vi "WebView2 Demo Browser.vi"() -> ()   [LabVIEW 2020]
uses:
  Webview2 Control/WebView2 Control.xctl
  Webview2 Control/Paths.ctl
panel:
  out "Paths":T1
  in  "stop":bool
  in  "FWD":bool
  in  "Back":bool
  out "Status":string
  out "navigation complete":bool
  in  "Reload":bool
  in  "Go":bool
  in  "URL":string="http://ni.com"
  out "WebView2 Browser Control":string(xcontrol)
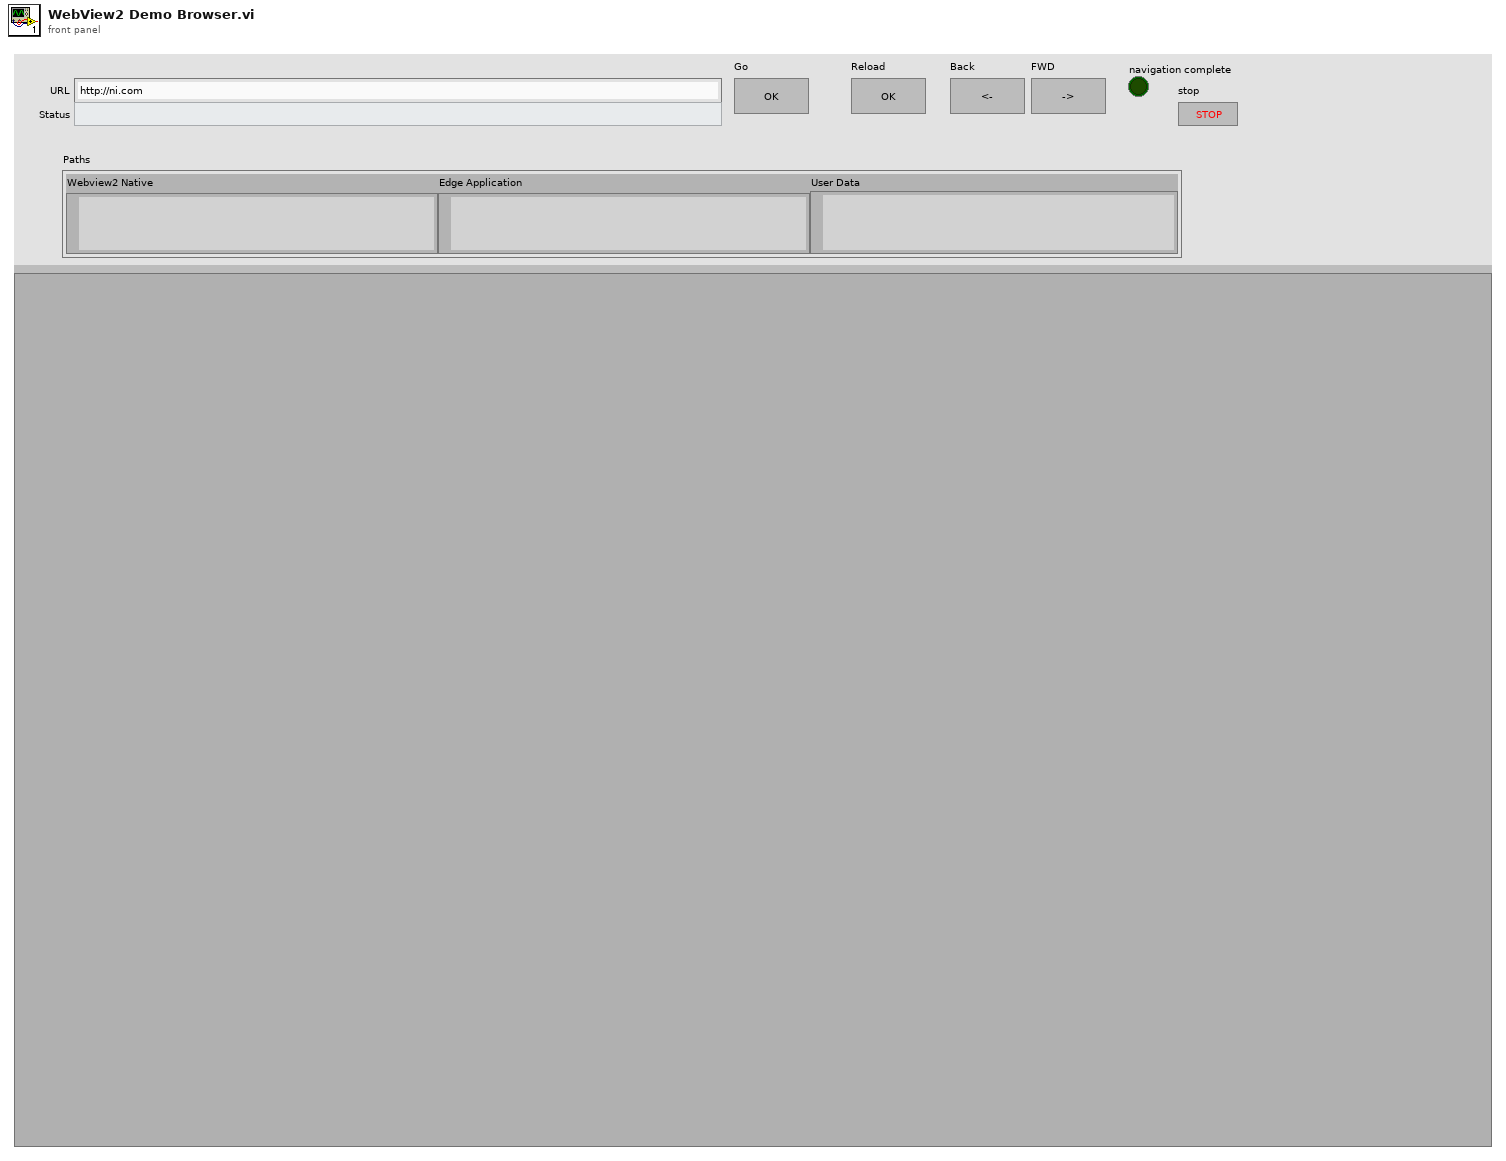
[diagram p1: front panel]
types:
  T1 = typedef "WebView2 Control.xctl/Paths.ctl" = cluster{"Webview2 Native":path, "Edge Application":path, "User Data":path}
  T2 = cluster{"Navigation Complete Event":refnum<user-event>, "Source Changed Event":refnum<user-event>, "Document Title Changed Event":refnum<user-event>, "Status Bar Text Changed":refnum<user-event>, "Web Message Received":refnum<user-event>, "Window Close Requested":refnum<user-event>}
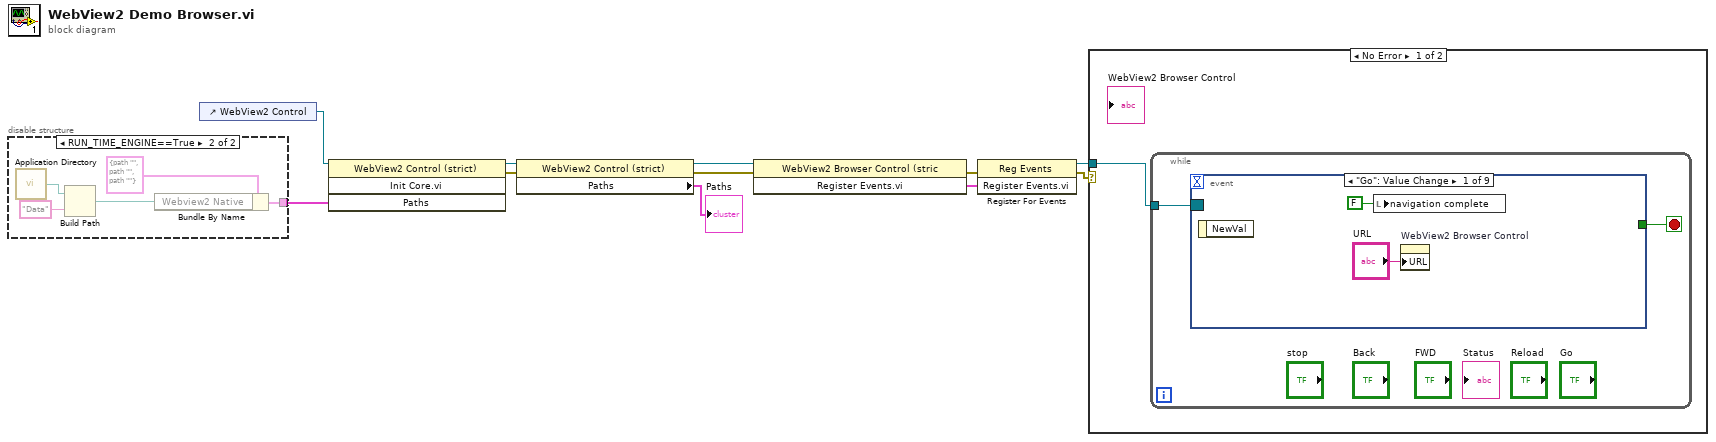
[diagram p0: block diagram]
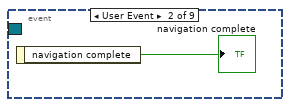
[diagram p3: hidden frame]
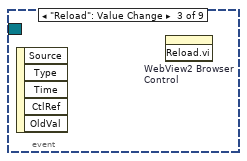
[diagram p4: hidden frame]
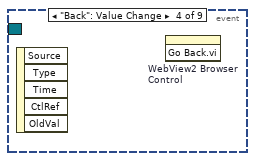
[diagram p5: hidden frame]
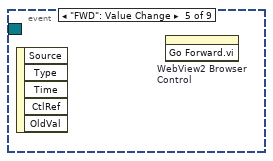
[diagram p6: hidden frame]
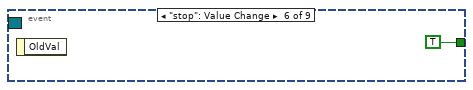
[diagram p7: hidden frame]
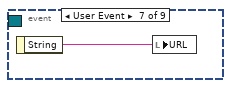
[diagram p8: hidden frame]
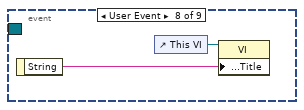
[diagram p9: hidden frame]
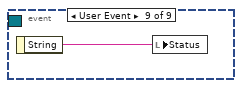
[diagram p10: hidden frame]
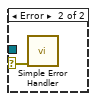
[diagram p11: hidden frame]
diagram:
  n1 = disable-structure shown="RUN_TIME_ENGINE==True" {
    disable-tunnel: [_ w15] -> w1
    frame condition #0 (active) {
    }
    frame condition #1 {
      n2 = call <vilib>:"Application Directory.vi"() -> ("Application Directory"=w13:path)
      n3 = Build Path(base path=w13, name or relative path="Data") -> (appended path=w14:path)
      n4 = Bundle By Name(cluster=T1 {"Webview2 Native"=path "", "Edge Application"=path "", "User Data"=path ""} ("Path Overrides"), "Webview2 Native"=w14) -> (w15:T1)
    }
  }
  n5 = control-ref of="WebView2 Control"() -> (w4:refnum<vi>)
  n6 = invoke class="WebView2 Control (strict)" method="Init Core.vi"(reference=w4, "Paths"=w1) -> (reference out=w3:refnum<vi>, error out=w2:errorcluster)  [unwired: 2 in, 2 out]
  n7 = property class="WebView2 Control (strict)"(reference=w3, error in=w2) -> (reference out=w9:refnum<vi>, error out=w8:errorcluster, "Paths"=→"Paths":T1)
  n8 = invoke class="WebView2 Browser Control (stric" method="Register Events.vi"(reference=w9, error in=w8) -> (error out=w6:errorcluster, "Register Events.vi"=w5:T2)  [unwired: 1 in, 1 out]
  n9 = register-events(error in=w6, w5) -> (reference out=w11:refnum<event-registration>, error out=w10:errorcluster)  [unwired: 1 in]
  n10 = case shown="No Error" w10 {
    selector: w10 -> [_ w28]
    tunnel: w11 -> [w17 _]
    frame No Error {
      n11 = while {
        tunnel: w17 -> [w19]
        stop <- w18 stop-if-true
        n12 = event shown="[0] \"Go\": Value Change" {
          selector: w19 -> [_ _ _ _ _ _ _ _ _]
          dyn-events: _ -> [_ _ _ _ _ _ _ _ _]
          timeout: _ -> [_ _ _ _ _ _ _ _ _]
          tunnel: [_ _ _ _ _ TRUE _ _ _] -> w18
          event "Go": Value Change {
            n13 = event-data() -> ()  [unwired: 1 in, 1 out]
            n14 = local write "navigation complete"(FALSE ("navigation complete")) -> ()
            n15 = property on="WebView2 Browser Control" class="WebView2 Control (strict)"("URL"="URL") -> ()  [unwired: 2 in, 2 out]
          }
          event User Event {
            n16 = event-data() -> ("navigation complete"=→"navigation complete":bool)  [unwired: 1 in]
          }
          event "Reload": Value Change {
            n17 = event-data() -> ()  [unwired: 1 in, 5 out]
            n18 = invoke on="WebView2 Browser Control" class="WebView2 Browser Control (stric" method="Reload.vi"() -> ()  [unwired: 3 in, 3 out]
          }
          event "Back": Value Change {
            n19 = event-data() -> ()  [unwired: 1 in, 5 out]
            n20 = invoke on="WebView2 Browser Control" class="WebView2 Browser Control (stric" method="Go Back.vi"() -> ()  [unwired: 3 in, 3 out]
          }
          event "FWD": Value Change {
            n21 = event-data() -> ()  [unwired: 1 in, 5 out]
            n22 = invoke on="WebView2 Browser Control" class="WebView2 Browser Control (stric" method="Go Forward.vi"() -> ()  [unwired: 3 in, 3 out]
          }
          event "stop": Value Change {
            n23 = event-data() -> ()  [unwired: 1 in, 1 out]
          }
          event User Event {
            n24 = event-data() -> ("String"=w24:string)  [unwired: 1 in]
            n25 = local write "URL"(w24) -> ()
          }
          event User Event {
            n26 = event-data() -> ("String"=w25:string)  [unwired: 1 in]
            n27 = control-ref of="This VI"() -> (w26:refnum<vi>)
            n28 = property class="VI"(reference=w26, "Front Panel.Title"=w25) -> ()  [unwired: 1 in, 2 out]
          }
          event User Event {
            n29 = event-data() -> ("String"=w27:string)  [unwired: 1 in]
            n30 = local write "Status"(w27) -> ()
          }
        }
      }
    }
    frame Error {
      n31 = call <vilib>:"Simple Error Handler.vi"("error in (no error)"=w28) -> ()  [unwired: 4 in, 5 out]
    }
  }
